vi "PCT FGV DATA Ref.vi"(7 "CMD":T2=enum."SET", 8 "error in (no error)":errorcluster) -> (0 "error out":errorcluster, 3 "Data REF":T1)   [LabVIEW 2020]
uses:
  PCT FGV CMD.ctl
  PCT Data REFs.ctl
  <instrlib>/PalmSens SDK for LabVIEW 5.10/PalmSens/MeasurementResults.ctl
  <instrlib>/PalmSens SDK for LabVIEW 5.10/PalmSens/LiveCurveResult.ctl
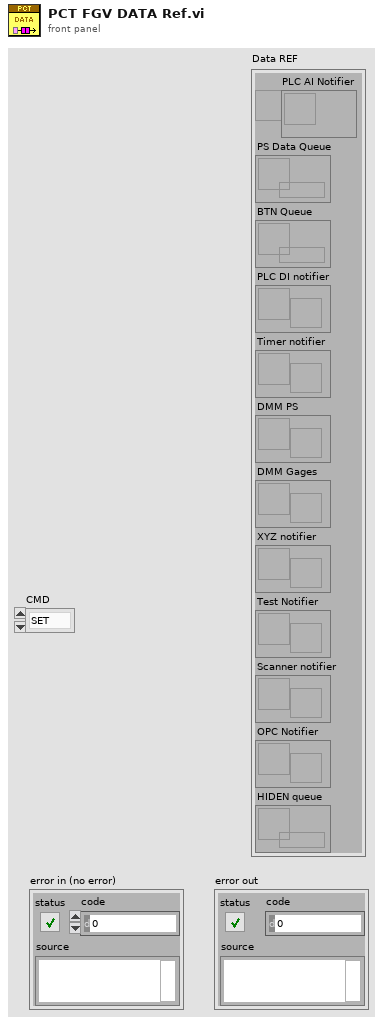
[diagram p1: front panel]
types:
  T1 = typedef "PCT Data REFs.ctl" = cluster{"PLC AI Notifier":refnum<notifier>, "PS Data Queue":refnum<queue>, "BTN Queue":refnum<queue>, "PLC DI notifier":refnum<notifier>, "Timer notifier":refnum<notifier>, "DMM PS":refnum<notifier>, "DMM Gages":refnum<notifier>, "XYZ notifier":refnum<notifier>, "Test Notifier":refnum<notifier>, "Scanner notifier":refnum<notifier>, "OPC Notifier":refnum<notifier>, "HIDEN queue":refnum<queue>}
  T2 = typedef "PCT FGV CMD.ctl" = enum16{"INIT", "GET", "SET"}
  T3 = typedef "MeasurementResults.ctl" = T4[]
  T4 = typedef "LiveCurveResult.ctl" = cluster{"X Label":string, "Y Label":string, "Name":string, "Index":i16, "Curve Values":cluster{"Values":cluster{"X Value":dbl, "Y Value":dbl}[], "Index":i16}}
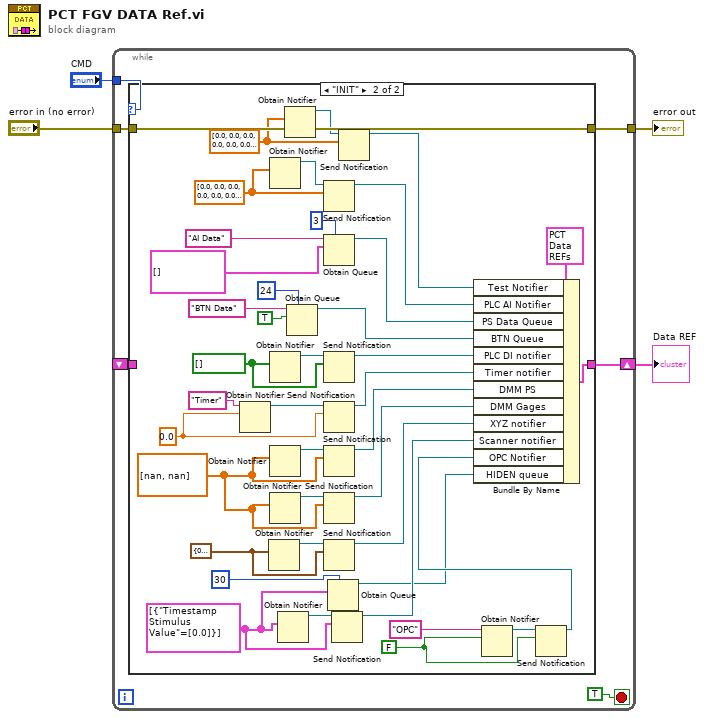
[diagram p0: block diagram]
diagram:
  n1 = while {
    tunnel: "CMD" -> [w8]
    shift-right: [w7] -> w1
    shift-left: _ -> [w6]
    tunnel: "error in (no error)" -> [w9]
    tunnel: [w10] -> w4
    stop <- TRUE stop-if-true
    n2 = case shown="\"INIT\"" w8 {
      tunnel: [w11 w51] -> w10
      tunnel: [w12 w52] -> w7
      tunnel: w9 -> [w11 w51]
      tunnel: w6 -> [w12 _]
      frame "GET", Default {
      }
      frame "INIT" {
        w15 = cluster{"Timestamp  Stimulus   Value":dbl[][]}[] [{"Timestamp  Stimulus   Value"=[[0.0]]}] ("Data out")
        w17 = cluster{"dX":dbl, "dY":dbl, "dZ":dbl, "dA":dbl} {"dX"=0.0, "dY"=0.0, "dZ"=0.0, "dA"=0.0} ("Axis Velocity")
        w18 = FALSE ("Boolean")
        w25 = dbl[] [nan, nan] ("register values")
        w28 = dbl[] [0.0, 0.0, 0.0, 0.0, 0.0, 0.0, 0.0, 0.0, 0.0, 0.0, 0.0, 0.0, 0.0, 0.0, 0.0, 0.0, 0.0, 0.0, 0.0] ("register values")
        w37 = 0.0 ("register")
        w39 = bool[] [] ("Boolean")
        w49 = dbl[] [0.0, 0.0, 0.0, 0.0, 0.0, 0.0, 0.0, 0.0, 0.0, 0.0, 0.0, 0.0, 0.0, 0.0, 0.0, 0.0, 0.0, 0.0, 0.0] ("register values")
        n3 = Obtain Notifier(name (unnamed)="Timer", notification data type=w37) -> (notifier out=w38:refnum<notifier>)  [unwired: 2 in, 2 out]
        n4 = Obtain Notifier(notification data type=w17) -> (notifier out=w30:refnum<notifier>)  [unwired: 3 in, 2 out]
        n5 = Obtain Notifier(notification data type=w49) -> (notifier out=w50:refnum<notifier>)  [unwired: 3 in, 2 out]
        n6 = Obtain Notifier(notification data type=w39) -> (notifier out=w41:refnum<notifier>)  [unwired: 3 in, 2 out]
        n7 = Obtain Notifier(notification data type=w25) -> (notifier out=w34:refnum<notifier>)  [unwired: 3 in, 2 out]
        n8 = Obtain Notifier(notification data type=w25) -> (notifier out=w33:refnum<notifier>)  [unwired: 3 in, 2 out]
        n9 = Obtain Notifier(notification data type=w15) -> (notifier out=w24:refnum<notifier>)  [unwired: 3 in, 2 out]
        n10 = Obtain Notifier(notification data type=w28) -> (notifier out=w27:refnum<notifier>)  [unwired: 3 in, 2 out]
        n11 = Obtain Queue(max queue size (-1, unlimited)=24, name (unnamed)="BTN Data", element data type=TRUE ("Boolean")) -> (queue out=w44:refnum<queue>)  [unwired: 2 in, 2 out]
        n12 = Send Notification(notification=w49, notifier=w50) -> (notifier out=w42:refnum<notifier>)  [unwired: 1 in, 1 out]
        n13 = Obtain Queue(max queue size (-1, unlimited)=3, name (unnamed)="AI Data", element data type=T3 [] ("Results")) -> (queue out=w47:refnum<queue>)  [unwired: 2 in, 2 out]
        n14 = Send Notification(notification=w39, notifier=w41) -> (notifier out=w40:refnum<notifier>)  [unwired: 1 in, 1 out]
        n15 = Send Notification(notification=w37, notifier=w38) -> (notifier out=w36:refnum<notifier>)  [unwired: 1 in, 1 out]
        n16 = Send Notification(notification=w25, notifier=w34) -> (notifier out=w32:refnum<notifier>)  [unwired: 1 in, 1 out]
        n17 = Send Notification(notification=w25, notifier=w33) -> (notifier out=w31:refnum<notifier>)  [unwired: 1 in, 1 out]
        n18 = Send Notification(notification=w17, notifier=w30) -> (notifier out=w29:refnum<notifier>)  [unwired: 1 in, 1 out]
        n19 = Obtain Queue(max queue size (-1, unlimited)=30, element data type=w15) -> (queue out=w14:refnum<queue>)  [unwired: 3 in, 2 out]
        n20 = Send Notification(notification=w15, notifier=w24) -> (notifier out=w23:refnum<notifier>)  [unwired: 1 in, 1 out]
        n21 = Send Notification(notification=w28, notifier=w27) -> (notifier out=w26:refnum<notifier>)  [unwired: 1 in, 1 out]
        n22 = Obtain Notifier(name (unnamed)="OPC", notification data type=w18) -> (notifier out=w21:refnum<notifier>)  [unwired: 2 in, 2 out]
        n23 = Send Notification(notification=w18, notifier=w21) -> (notifier out=w19:refnum<notifier>)  [unwired: 1 in, 1 out]
        n24 = Bundle By Name(cluster=T1 {"PLC AI Notifier"=refnum, "PS Data Queue"=refnum, "BTN Queue"=refnum, "PLC DI notifier"=refnum, "Timer notifier"=refnum, "DMM PS"=refnum, "DMM Gages"=refnum, "XYZ notifier"=refnum, "Test Notifier"=refnum, "Scanner notifier"=refnum, "OPC Notifier"=refnum, "HIDEN queue"=refnum} ("Data REF"), "Test Notifier"=w26, "PLC AI Notifier"=w42, "PS Data Queue"=w47, "BTN Queue"=w44, "PLC DI notifier"=w40, "Timer notifier"=w36, "DMM PS"=w32, "DMM Gages"=w31, "XYZ notifier"=w29, "Scanner notifier"=w23, "OPC Notifier"=w19, "HIDEN queue"=w14) -> (w52:T1)
      }
    }
  }
  "error out" <- w4
  "Data REF" <- w1
